vi "Main.vi"() -> ()   [LabVIEW 2020]
doc: "Chronomètre"
uses:
  Ctrl/Ctrl_states.ctl
panel:
  out "Time ?":bool
  out "Standard":cluster{"Minute":dbl, "Seconde":dbl}
  out "Countdown":dbl
  out "Pause TimeTime":dbl
  out "Time":dbl
  in  "Taget Time":dbl format="%#_g s"
  in  "FGV_state":T1
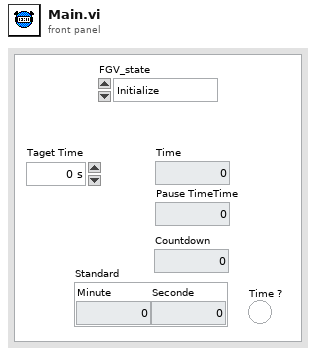
[diagram p1: front panel]
types:
  T1 = typedef "Ctrl_states.ctl" = enum16{"Initialize", "Time", "Pause"}
  T2 = typedef "Ctrl_Local.ctl" = cluster{"Initial Tick":u32, "Tick Time":u32, "Tick Pause":u32, "Time":dbl, "Pause TimeTime":dbl, "Previous Pause TimeTime":dbl, "Countdown":dbl, "Standard":cluster{"Minute":dbl, "Seconde":dbl}, "Time ?":bool}
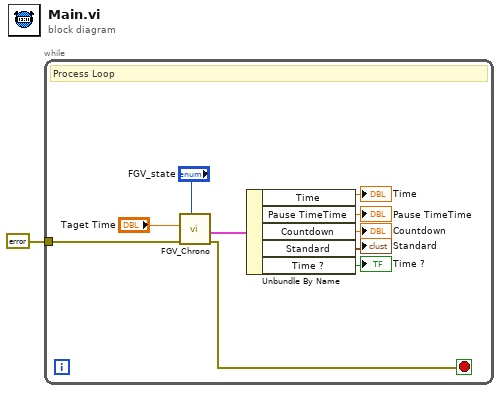
[diagram p0: block diagram]
diagram:
  n1 = while {
    tunnel: errorcluster {"status"=FALSE, "code"=0, "source"=""} ("error in") -> [w7]
    stop <- w8 stop-if-true
    # "Process Loop"
    n2 = call "FGV_Chrono.vi"("FGV_state"="FGV_state", "error in"=w7, "Taget Time"="Taget Time") -> ("error out"=w8:errorcluster, "Local"=w10:T2)  [unwired: 7 in]
    n3 = Unbundle By Name(w10) -> ("Time"=→"Time":dbl, "Pause TimeTime"=→"Pause TimeTime":dbl, "Countdown"=→"Countdown":dbl, "Standard"=→"Standard":cluster{"Minute":dbl, "Seconde":dbl}, "Time ?"=→"Time ?":bool)
  }
